vi "Timer.vi"(8 "error in (no error)":errorcluster, 9 "Time Target(s)":dbl, 10 "Reset":bool, 11 "Pause":bool) -> (0 "error out":errorcluster, 1 "Elapsed Time":dbl, 2 "Elapsed?":bool)   [LabVIEW 2013]
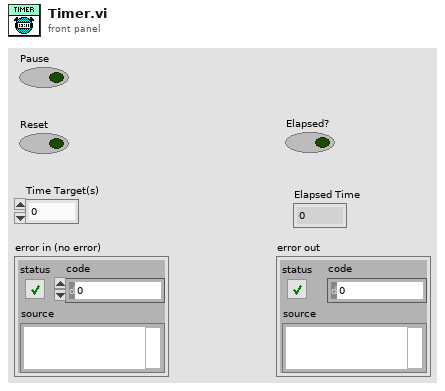
[diagram p1: front panel]
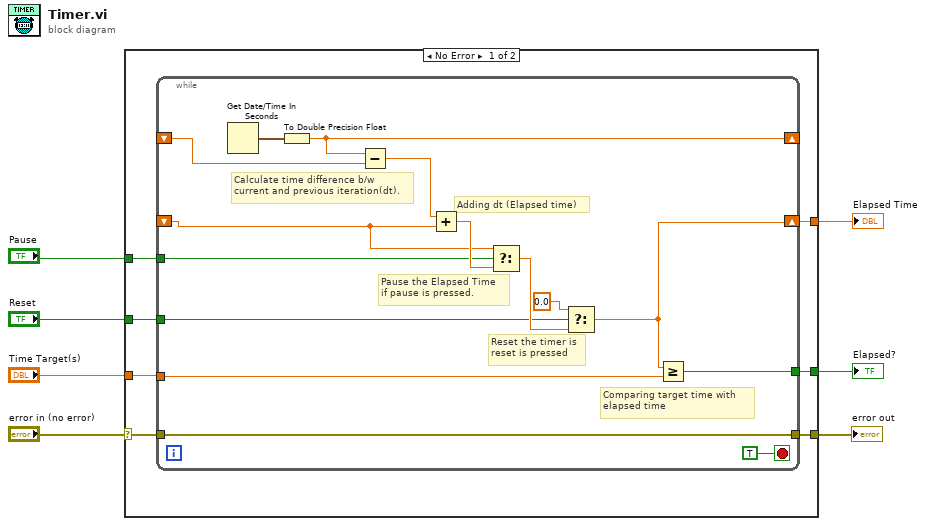
[diagram p0: block diagram]
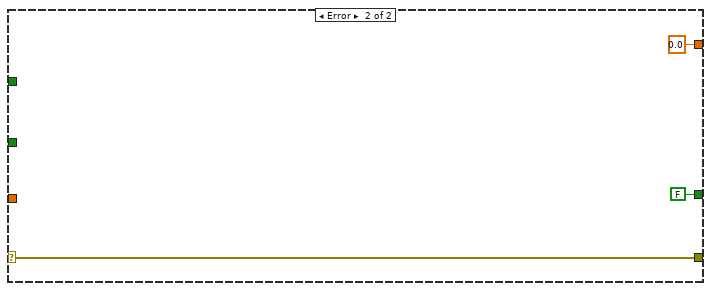
[diagram p2: hidden frame]
diagram:
  n1 = case shown="No Error" "error in (no error)" {
    selector: "error in (no error)" -> [w8 w32]
    tunnel: "Pause" -> [w14 _]
    tunnel: "Reset" -> [w13 _]
    tunnel: "Time Target(s)" -> [w12 _]
    tunnel: [w11 0.0 ("t")] -> w4
    tunnel: [w10 FALSE] -> w5
    tunnel: [w9 w32] -> w7
    frame No Error {
      n2 = while {
        shift-right: [w27] -> _
        shift-left: _ -> [w28]
        shift-right: [w18] -> w11
        shift-left: _ -> [w24]
        tunnel: w14 -> [w23]
        tunnel: w13 -> [w20]
        tunnel: w12 -> [w19]
        tunnel: [w17] -> w10
        tunnel: [w16] -> w9
        tunnel: w8 -> [w16]
        stop <- TRUE stop-if-true
        # "Comparing target time with \nelapsed time"
        # "Reset the timer is \nreset is pressed"
        # "Pause the Elapsed Time \nif pause is pressed."
        # "Adding dt (Elapsed time)"
        # "Calculate time difference b/w \ncurrent and previous iteration(dt)."
        n3 = Get Date/Time In Seconds() -> (seconds since 1Jan1904=w29:timestamp)
        n4 = To Double Precision Float(number=w29) -> (double precision float=w27:dbl)
        n5 = Subtract(x=w27, y=w28) -> (x-y=w26:dbl)
        n6 = Add(x=w26, y=w24) -> (x+y=w25:dbl)
        n7 = Select(t=w24, s=w23, f=w25) -> (s? t:f=w22:dbl)
        n8 = Select(t=0.0, s=w20, f=w22) -> (s? t:f=w18:dbl)
        n9 = Greater Or Equal?(x=w18, y=w19) -> (x >= y?=w17:bool)
      }
    }
    frame Error {
    }
  }
  "error out" <- w7
  "Elapsed?" <- w5
  "Elapsed Time" <- w4
